vi "TE_Alarm_Test.vi"() -> ()   [LabVIEW 2018]
panel:
  out "Temps":dbl[](array[numeric])
  in  "SendData":i32
  in  "WriteCommand":string="01"
  in  "ReadCommand":string="01"
  out "error out":errorcluster
  out "Response":dbl[](array[numeric])
  in  "Address":string[](array[string])=["01", "02", "03"]
  in  "Port":refnum<visa-resource-name>="Port1"
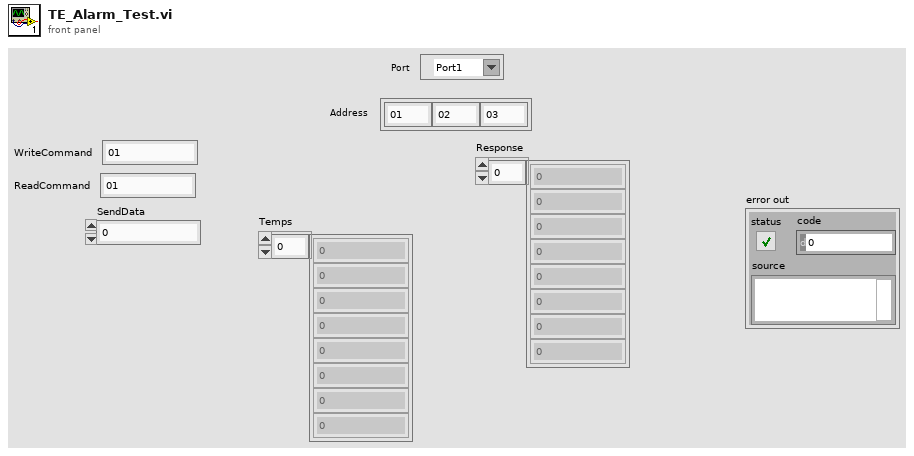
[diagram p1: front panel]
types:
  T1 = cluster{"port":refnum<visa-resource-name>, "timeout":u32, "baud":u32, "dataBits":u16, "stopBits":u16, "flowControl":u16, "parity":u16, "termChar":bool, "checkSum":bool, "checkSumVal":string}
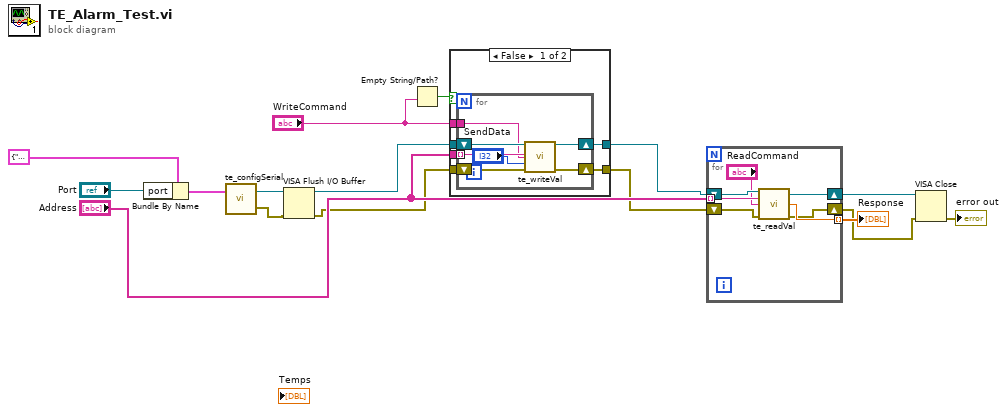
[diagram p0: block diagram]
diagram:
  n1 = Bundle By Name(cluster=T1 {"port"="COM1", "timeout"=4000, "baud"=115200, "dataBits"=8, "stopBits"=10, "flowControl"=0, "parity"=0, "termChar"=FALSE, "checkSum"=FALSE, "checkSumVal"=""} ("teSerial"), "port"="Port") -> (w15:T1)
  n2 = call "te_configSerial.vi"("teSerial"=w15) -> ("error out"=w10:errorcluster, "VISA resource name out"=w14:refnum<visa-resource-name>)  [unwired: 1 in]
  n3 = VISA Flush I/O Buffer(VISA resource name=w14, error in (no error)=w10) -> (VISA resource name out=w7:refnum<visa-resource-name>, error out=w4:errorcluster)  [unwired: 1 in]
  n4 = Empty String/Path?(string/path="WriteCommand") -> (empty?=w2:bool)
  n5 = case shown="False" w2 {
    tunnel: w7 -> [w22 w30]
    tunnel: [w21 w30] -> w6
    tunnel: "Address" -> [w20 _]
    tunnel: w4 -> [w19 w31]
    tunnel: [w18 w31] -> w3
    tunnel: "WriteCommand" -> [w17 _]
    frame False {
      n6 = for {
        tunnel: w20 -> [w27] mode=indexing
        shift-right: [w28] -> w21
        shift-left: w22 -> [w29]
        shift-right: [w25] -> w18
        shift-left: w19 -> [w26]
        tunnel: w17 -> [w24]
        n7 = call "te_writeVal.vi"("VISA In"=w29, "Hex Address"=w27, "Command"=w24, "Data"="SendData", "Error In"=w26) -> ("VISA Out"=w28:refnum<visa-resource-name>, "error out"=w25:errorcluster)  [unwired: 7 in, 2 out]
      }
    }
    frame True {
      # "Nothing to send"
    }
  }
  n8 = for {
    tunnel: "Address" -> [w36] mode=indexing
    shift-right: [w37] -> w12
    shift-left: w6 -> [w38]
    tunnel: [w35] -> w11 mode=indexing
    shift-right: [w33] -> w9
    shift-left: w3 -> [w34]
    n9 = call "te_readVal.vi"("VISA In"=w38, "Hex Address"=w36, "Command"="ReadCommand", "Error In"=w34) -> ("VISA Out"=w37:refnum<visa-resource-name>, "Response"=w35:dbl, "error out"=w33:errorcluster)  [unwired: 7 in, 2 out]
  }
  "Response" <- w11
  n10 = VISA Close(VISA resource name=w12, error in (no error)=w9) -> (error out=→"error out":errorcluster)
